vi "Manage Scan Info File.vi"(7 "CONFIGURATION CLUSTER IN":T1, 8 "SAVE MODE":enum16{"DO NOT SAVE", "SAVE .CNF FILE"}(ring), 9 "PROCESSING MODE":T3(ring), 11 "SCAN INFO CLUSTER ARRAY IN":T2(array[cluster]) {"SCAN ENABLED" items=["NO", "YES"]; "INPUT" items=["ZERO", "MEAS", "CAL"]; "RANGE" items=["NO RANGE", "2 Ohms", "20 Ohms", "200 Ohms", "2 kOhms", "20 kOhms", "200 kOhms", "2 MOhms"]; "AUTORANGE" items=["NO", "YES"]; "EXCITATION" items=["NO EXCITATION", "3 uV", "10uV", "30uV", "100uV", "300uV", "1mV", "3mV"]}) -> (1 "SCAN FILE READ INFO":string, 3 "SCAN INFO CLUSTER ARRAY OUT":T2(array[cluster])=[{"SCAN ENABLED"=0, "INPUT"=0, "RANGE"=3, "AUTORANGE"=0, "EXCITATION"=0, "STAB DELAY"=0, "AVERAGE COUNT"=1}, {"SCAN ENABLED"=0, "INPUT"=0, "RANGE"=3, "AUTORANGE"=0, "EXCITATION"=0, "STAB DELAY"=0, "AVERAGE COUNT"=1}, {"SCAN ENABLED"=0, "INPUT"=0, "RANGE"=3, "AUTORANGE"=0, "EXCITATION"=0, "STAB DELAY"=0, "AVERAGE COUNT"=1}, {"SCAN ENABLED"=0, "INPUT"=0, "RANGE"=3, "AUTORANGE"=0, "EXCITATION"=0, "STAB DELAY"=0, "AVERAGE COUNT"=1}, {"SCAN ENABLED"=0, "INPUT"=0, "RANGE"=3, "AUTORANGE"=0, "EXCITATION"=0, "STAB DELAY"=0, "AVERAGE COUNT"=1}, {"SCAN ENABLED"=0, "INPUT"=0, "RANGE"=3, "AUTORANGE"=0, "EXCITATION"=0, "STAB DELAY"=0, "AVERAGE COUNT"=1}, {"SCAN ENABLED"=0, "INPUT"=0, "RANGE"=3, "AUTORANGE"=0, "EXCITATION"=0, "STAB DELAY"=0, "AVERAGE COUNT"=1}, {"SCAN ENABLED"=0, "INPUT"=0, "RANGE"=3, "AUTORANGE"=0, "EXCITATION"=0, "STAB DELAY"=0, "AVERAGE COUNT"=1}] {"SCAN ENABLED" items=["NO", "YES"]; "INPUT" items=["ZERO", "MEAS", "CAL"]; "RANGE" items=["NO RANGE", "2 Ohms", "20 Ohms", "200 Ohms", "2 kOhms", "20 kOhms", "200 kOhms", "2 MOhms"]; "AUTORANGE" items=["NO", "YES"]; "EXCITATION" items=["NO EXCITATION", "3 uV", "10uV", "30uV", "100uV", "300uV", "1mV", "3mV"]}, 5 "CONFIGURATION CLUSTER OUT":T1)   [LabVIEW 2012]
doc: "Read, edit and save the Scan Info File.\nScan Info File specifies the settings that\nare used for each scan-enabled channel in\na scanner application."
uses:
  <vilib>/Utility/error.llb/DialogType.ctl
panel:
  in  "EDIT INFO":T2(array[cluster])=[{"SCAN ENABLED"=0, "INPUT"=0, "RANGE"=3, "AUTORANGE"=0, "EXCITATION"=0, "STAB DELAY"=0, "AVERAGE COUNT"=1}, {"SCAN ENABLED"=0, "INPUT"=0, "RANGE"=3, "AUTORANGE"=0, "EXCITATION"=0, "STAB DELAY"=0, "AVERAGE COUNT"=1}, {"SCAN ENABLED"=0, "INPUT"=0, "RANGE"=3, "AUTORANGE"=0, "EXCITATION"=0, "STAB DELAY"=0, "AVERAGE COUNT"=1}, {"SCAN ENABLED"=0, "INPUT"=0, "RANGE"=3, "AUTORANGE"=0, "EXCITATION"=0, "STAB DELAY"=0, "AVERAGE COUNT"=1}, {"SCAN ENABLED"=0, "INPUT"=0, "RANGE"=3, "AUTORANGE"=0, "EXCITATION"=0, "STAB DELAY"=0, "AVERAGE COUNT"=1}, {"SCAN ENABLED"=0, "INPUT"=0, "RANGE"=3, "AUTORANGE"=0, "EXCITATION"=0, "STAB DELAY"=0, "AVERAGE COUNT"=1}, {"SCAN ENABLED"=0, "INPUT"=0, "RANGE"=3, "AUTORANGE"=0, "EXCITATION"=0, "STAB DELAY"=0, "AVERAGE COUNT"=1}, {"SCAN ENABLED"=0, "INPUT"=0, "RANGE"=3, "AUTORANGE"=0, "EXCITATION"=0, "STAB DELAY"=0, "AVERAGE COUNT"=1}] {"SCAN ENABLED" items=["NO", "YES"]; "INPUT" items=["ZERO", "MEAS", "CAL"]; "RANGE" items=["NO RANGE", "2 Ohms", "20 Ohms", "200 Ohms", "2 kOhms", "20 kOhms", "200 kOhms", "2 MOhms"]; "AUTORANGE" items=["NO", "YES"]; "EXCITATION" items=["NO EXCITATION", "3 uV", "10uV", "30uV", "100uV", "300uV", "1mV", "3mV"]}
  in  "DISCARD":bool
  in  "ACCEPT":bool
  out "FILE READ INFO":string
  out "INFO STRING 1":string
  # "Manage Scan Info File.vi"
  # "Scan setting can be \nedited after this VI has\nbeen started  in the \n\"read and edit\" \nprocessing mode."
  # "AND PROCEED"
  # "This VI has four processing modes and two save modes:\n1. NONE:  The input Scan Info Cluster goes transparently through the VI.\n                   The cluster can be saved/not saved.\n2. READ: The  \"avs47b_scan_info.cnf\" file is read from the operating \n                   directory, and is the output of the VI.  The output cluster can\n                    be saved, but as there are no changes in this case, saving is\n                    not meaningful. If the information file is not found or is \n                    invalid, a default cluster is used instead. The default settings\n                    must be edited in order to be useful.\n3.  READ AND EDIT: The information file is read and settings for any or\n                    all of the 8 channels can be edited by selecting values in\n                    the \"SCAN INFO\" array. Once ready, choose either to accept\n                    or discard the edits and the VI proceeds to the next step,\n                    which is to save or not to save the settings, depending on\n                    the selected save mode. \n                            Because the VI stops for editing, this processing mode\n                     is not suitable for programmatic use. It can, however,  be\n                     used as such for creating an info file with useful settings.\n4. DEFAULTS:  The output is a default scan info cluster, which can be\n                      saved/not saved depending on the save settings.  The VI\n                       does not try to read the disk file."
  # "If this VI does not find the file  Avs47b_scan_info.cnf in the operating\ndirectory, it creates a default file, which you must then edit according\nto your experimental setup. Use \"Scanner with R and T displays.vi\"\nfor editing and saving the information file.\n\nThis information file specifies whether a channel is included in the\nscan cycle or not, the position of the input switch,  measuring range\n(or initial range, if autoranging is enabled),  autoranging enabled/disabled\nfor this channel, excitation, stabilisation delay and average count for\nthis channel."
  # "SCAN INFO"
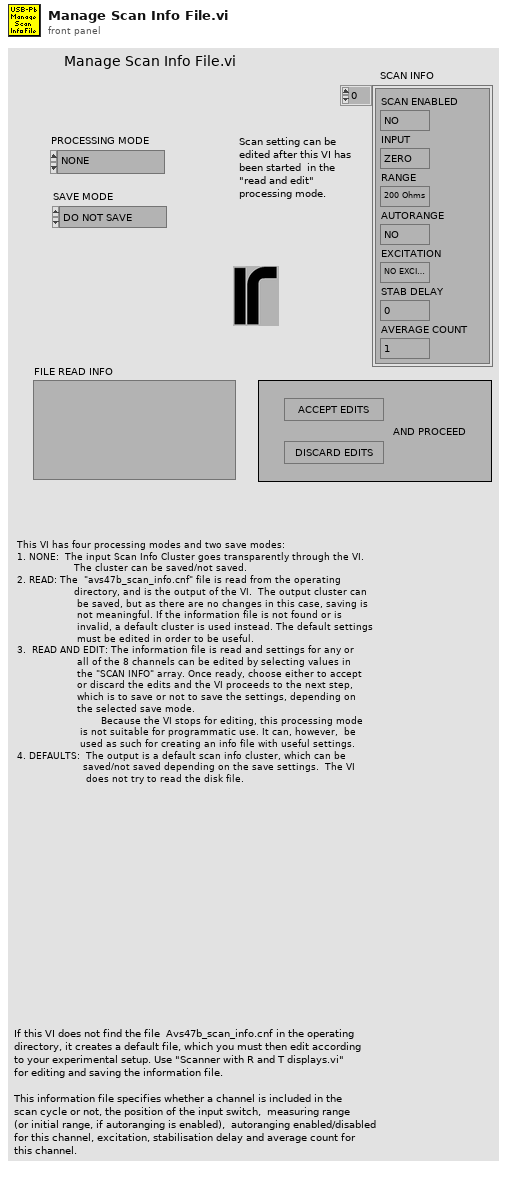
[diagram p1: front panel]
types:
  T1 = cluster{"VISA RESOURCE":refnum<visa-resource-name>, "PICOBUS ADDRESS":u8, "DISABLE AL":u8, "REMOTE":u8, "INPUT":u8, "CHANNEL":u8, "RANGE":u8, "EXCITATION":u8, "DISPLAY":u8, "DIGITAL REFERENCE":u16, "SET POINT":dbl, "PROP GAIN":u8, "INTG":u8, "DERIV":u8, "POWER BIAS":u8, "POWER RANGE":u8, "INFO STRING":string, "HEATER RESISTANCE":dbl, "INTERVAL":u8, " SENSOR dR/dT":u8}
  T2 = cluster{"SCAN ENABLED":u8, "INPUT":u8, "RANGE":u8, "AUTORANGE":u8, "EXCITATION":u8, "STAB DELAY":i32, "AVERAGE COUNT":i32}[]
  T3 = enum16{"NONE", "READ", "READ AND EDIT", "DEFAULTS"}
  T4 = cluster{"SCAN ENABLED":u8, "INPUT":u8, "RANGE":u8, "AUTORANGE":u8, "EXCITATION":u8, "STAB DELAY":i32, "AVERAGE COUNT":i32}
  T5 = enum16{"open", "replace", "create", "open or create", "replace or create", "replace or create with confirmation"}
  T6 = typedef "DialogType.ctl" = u16
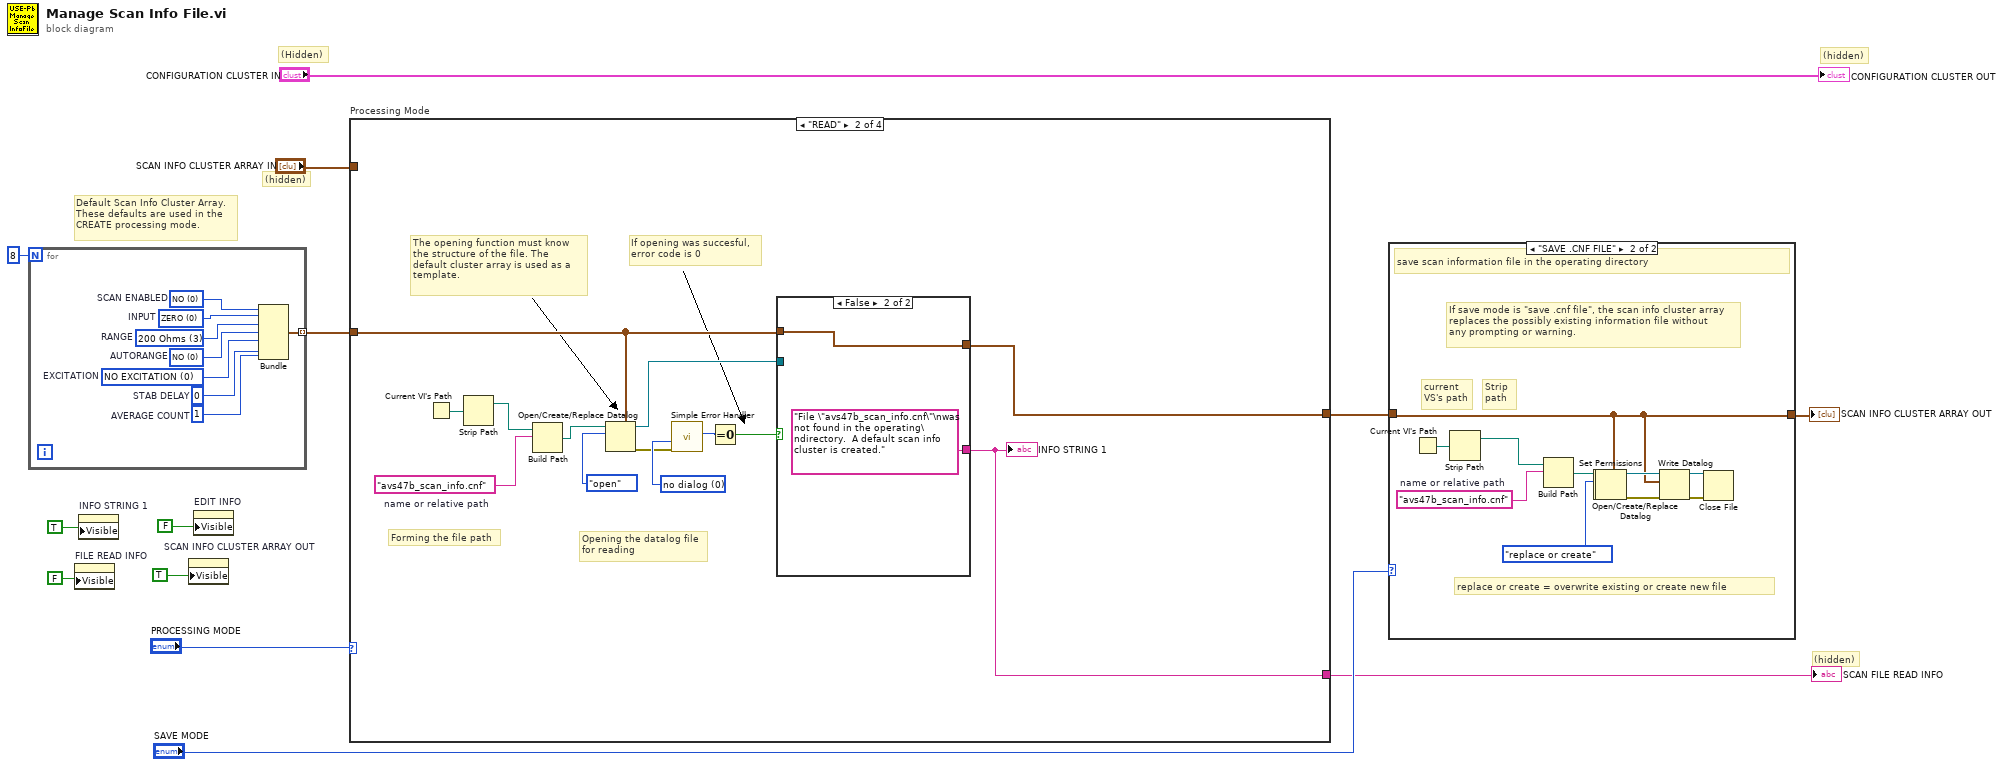
[diagram p0: block diagram]
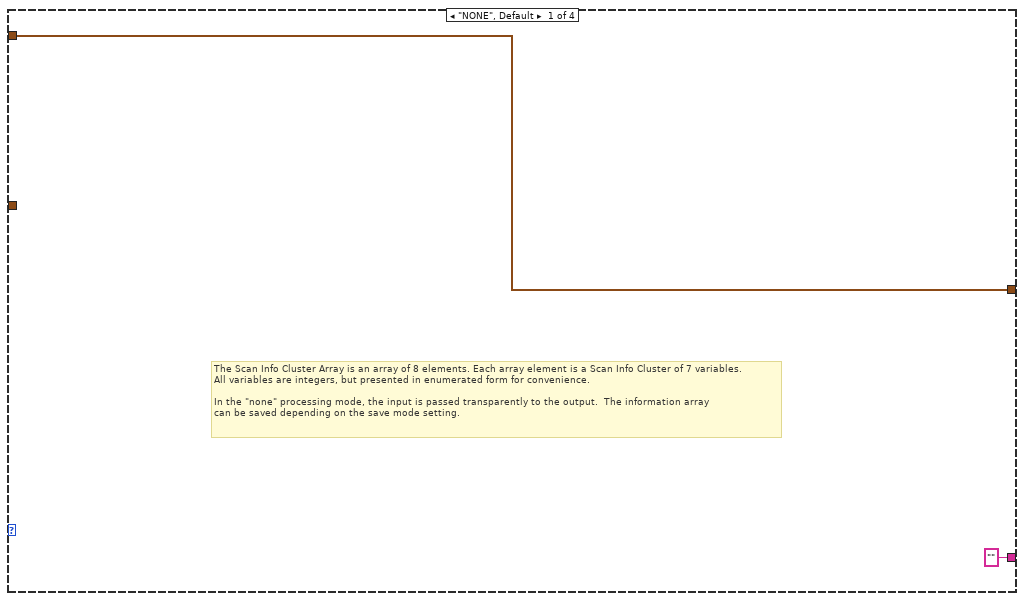
[diagram p3: hidden frame]
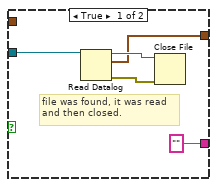
[diagram p4: hidden frame]
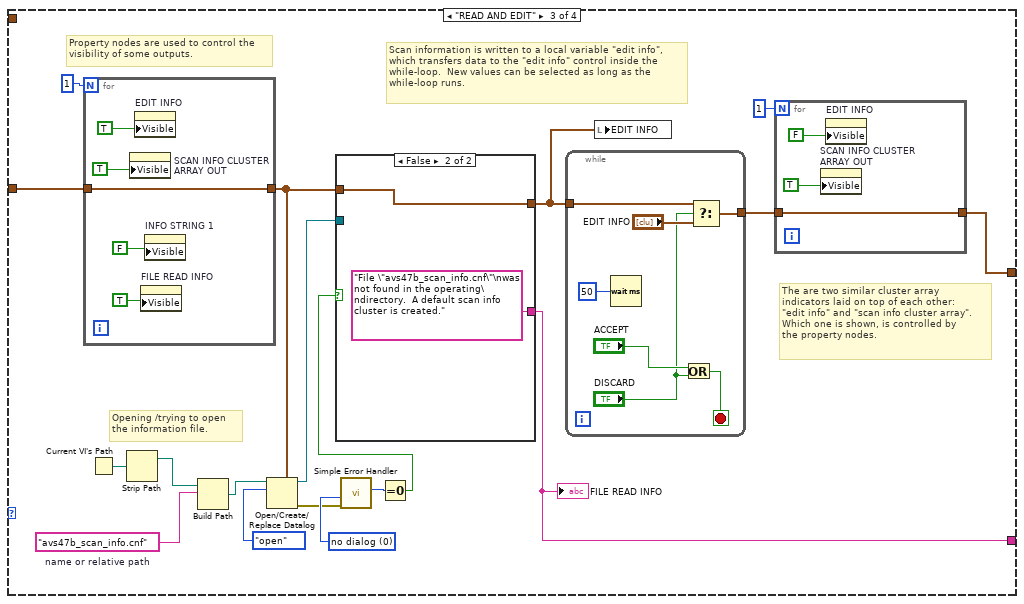
[diagram p5: hidden frame]
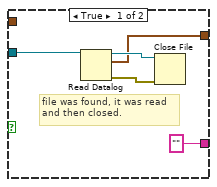
[diagram p6: hidden frame]
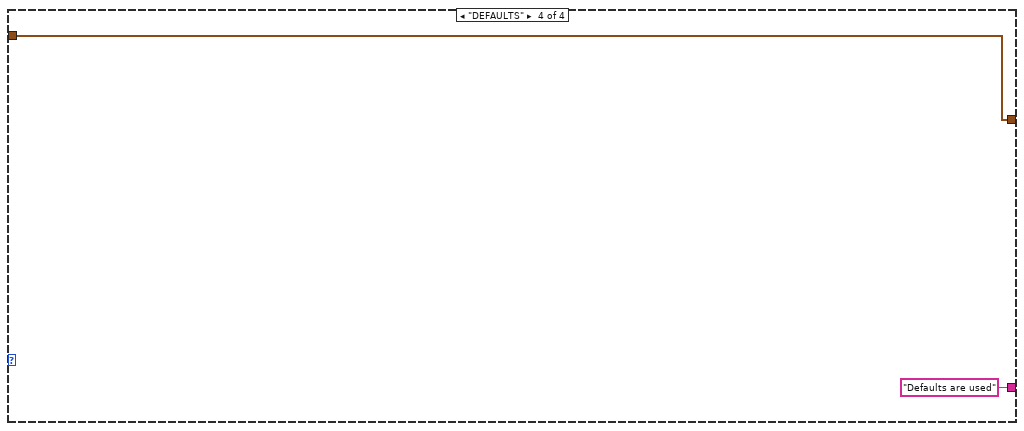
[diagram p7: hidden frame]
diagram:
  # "(Hidden)"
  # "(hidden)"
  # "(hidden)"
  # "(hidden)"
  # "Default Scan Info Cluster Array.\nThese defaults are used in the\nCREATE processing mode."
  n1 = for {
    N: 8 -> [_]
    tunnel: [w14] -> w12 mode=indexing
    w15 = 1  # AVERAGE COUNT
    w16 = 0  # STAB DELAY
    w17 = u8 0 items=["NO EXCITATION", "3 uV", "10uV", "30uV", "100uV", "300uV", "1mV", "3mV"]  # EXCITATION
    w18 = u8 0 items=["NO", "YES"]  # AUTORANGE
    w19 = u8 3 items=["NO RANGE", "2 Ohms", "20 Ohms", "200 Ohms", "2 kOhms", "20 kOhms", "200 kOhms", "2 MOhms"]  # RANGE
    w20 = u8 0 items=["ZERO", "MEAS", "CAL"]  # INPUT
    w21 = u8 0 items=["NO", "YES"]  # SCAN ENABLED
    n2 = Bundle("SCAN ENABLED"=w21, "INPUT"=w20, "RANGE"=w19, "AUTORANGE"=w18, "EXCITATION"=w17, "STAB DELAY"=w16, "AVERAGE COUNT"=w15) -> (w14:T4)  [unwired: 1 in]
  }
  n3 = property on="FILE READ INFO" class="Str"("Visible"=FALSE) -> ()  [unwired: 2 in, 2 out]
  n4 = property on="INFO STRING 1" class="Str"("Visible"=TRUE) -> ()  [unwired: 2 in, 2 out]
  n5 = property on="SCAN INFO CLUSTER ARRAY OUT" class="Arr (strict)"("Visible"=TRUE) -> ()  [unwired: 2 in, 2 out]
  n6 = property on="EDIT INFO" class="Arr (strict)"("Visible"=FALSE) -> ()  [unwired: 2 in, 2 out]
  n7 = case "Processing Mode" shown="\"READ\"" "PROCESSING MODE" {
    tunnel: w12 -> [_ w28 w50 w85]
    tunnel: "SCAN INFO CLUSTER ARRAY IN" -> [w23 _ _ _]
    tunnel: [w23 w25 w47 w85] -> w5
    tunnel: ["" w24 w44 "Defaults are used"] -> w2
    frame "NONE", Default {
      # "The Scan Info Cluster Array is an array of 8 elements. Each array element is a Scan Info Cluster of 7 variables.\nAll variables are integers, but presented in enumerated form for convenience.\n\nIn the \"none\" processing mode, the input is passed transparently to the output.  The information array\ncan be saved depending on the save mode setting."
    }
    frame "READ" {
      w34 = T6 0 items=["no dialog", "OK message", "continue or stop message", "OK message + warnings", "continue/stop + warnings"] ("type of dialog (OK msg:1)")
      w30 = "avs47b_scan_info.cnf"  # name or relative path
      # "The opening function must know\nthe structure of the file. The \ndefault cluster array is used as a \ntemplate."
      # "If opening was succesful,\nerror code is 0"
      # "Opening the datalog file\nfor reading"
      # "Forming the file path"
      n8 = Current VI's Path() -> (path=w31:path)
      n9 = Strip Path(path=w31) -> (stripped path=w32:path)  [unwired: 1 out]
      n10 = Build Path(base path=w32, name or relative path=w30) -> (appended path=w27:path)
      n11 = Open/Create/Replace Datalog(5:w28, 10:T5."open" ("operation (0:open)"), 11:w27) -> (0:w33:errorcluster, 3:w26:refnum<k1>)  [unwired: 3 in, 1 out]
      n12 = call <vilib>:"Simple Error Handler.vi"("type of dialog (OK msg:1)"=w34, "error in (no error)"=w33) -> ("code out"=w36:i32)  [unwired: 3 in, 4 out]
      n13 = Equal To 0?(x=w36) -> (x = 0?=w29:bool)
      n14 = case shown="False" w29 {
        tunnel: w28 -> [_ w43]
        tunnel: [w39 w43] -> w25
        tunnel: ["" "File \"avs47b_scan_info.cnf\"\nwas not found in the operating\ndirectory.  A default scan info cluster is created."] -> w24
        tunnel: w26 -> [w37 _]
        frame True {
          # "file was found, it was read\nand then closed."
          n15 = Read Datalog(7:w37) -> (0:w41:errorcluster, 2:w39:T2, 3:w40:refnum<k1>)  [unwired: 2 in]
          n16 = Close File(refnum=w40, error in=w41) -> ()  [unwired: 2 out]
        }
        frame False {
        }
      }
      "INFO STRING 1" <- w24
    }
    frame "READ AND EDIT" {
      w59 = T6 0 items=["no dialog", "OK message", "continue or stop message", "OK message + warnings", "continue/stop + warnings"] ("type of dialog (OK msg:1)")
      w55 = "avs47b_scan_info.cnf"  # name or relative path
      # "The are two similar cluster array\nindicators laid on top of each other:\n\"edit info\" and \"scan info cluster array\".\nWhich one is shown, is controlled by\nthe property nodes."
      # "Scan information is written to a local variable \"edit info\",\nwhich transfers data to the \"edit info\" control inside the\nwhile-loop.  New values can be selected as long as the\nwhile-loop runs."
      # "Opening /trying to open\nthe information file."
      # "Property nodes are used to control the\nvisibility of some outputs."
      n17 = for {
        N: 1 -> [_]
        tunnel: w50 -> [w67]
        tunnel: [w67] -> w49
        n18 = property on="SCAN INFO CLUSTER ARRAY OUT" class="Arr (strict)"("Visible"=TRUE) -> ()  [unwired: 2 in, 2 out]
        n19 = property on="EDIT INFO" class="Arr (strict)"("Visible"=TRUE) -> ()  [unwired: 2 in, 2 out]
        n20 = property on="FILE READ INFO" class="Str"("Visible"=TRUE) -> ()  [unwired: 2 in, 2 out]
        n21 = property on="INFO STRING 1" class="Str"("Visible"=FALSE) -> ()  [unwired: 2 in, 2 out]
      }
      n22 = Current VI's Path() -> (path=w56:path)
      n23 = Strip Path(path=w56) -> (stripped path=w57:path)  [unwired: 1 out]
      n24 = Build Path(base path=w57, name or relative path=w55) -> (appended path=w53:path)
      n25 = Open/Create/Replace Datalog(5:w49, 10:T5."open" ("operation (0:open)"), 11:w53) -> (0:w58:errorcluster, 3:w52:refnum<k1>)  [unwired: 3 in, 1 out]
      n26 = call <vilib>:"Simple Error Handler.vi"("type of dialog (OK msg:1)"=w59, "error in (no error)"=w58) -> ("code out"=w61:i32)  [unwired: 3 in, 4 out]
      n27 = Equal To 0?(x=w61) -> (x = 0?=w54:bool)
      n28 = case shown="False" w54 {
        tunnel: w49 -> [_ w83]
        tunnel: [w79 w83] -> w51
        tunnel: ["" "File \"avs47b_scan_info.cnf\"\nwas not found in the operating\ndirectory.  A default scan info cluster is created."] -> w44
        tunnel: w52 -> [w77 _]
        frame True {
          # "file was found, it was read\nand then closed."
          n29 = Read Datalog(7:w77) -> (0:w81:errorcluster, 2:w79:T2, 3:w80:refnum<k1>)  [unwired: 2 in]
          n30 = Close File(refnum=w80, error in=w81) -> ()  [unwired: 2 out]
        }
        frame False {
        }
      }
      "FILE READ INFO" <- w44
      n31 = while {
        tunnel: w51 -> [w73]
        tunnel: [w70] -> w48
        stop <- w74 stop-if-true
        n32 = Wait (ms)(milliseconds to wait=u32 50) -> ()  [unwired: 1 out]
        n33 = Or(x="ACCEPT", y="DISCARD") -> (x .or. y?=w74:bool)
        n34 = Select(t=w73, s="DISCARD", f="EDIT INFO") -> (s? t:f=w70:T2)
      }
      n35 = local write "EDIT INFO"(w51) -> ()
      n36 = for {
        N: 1 -> [_]
        tunnel: w48 -> [w62]
        tunnel: [w62] -> w47
        n37 = property on="SCAN INFO CLUSTER ARRAY OUT" class="Arr (strict)"("Visible"=TRUE) -> ()  [unwired: 2 in, 2 out]
        n38 = property on="EDIT INFO" class="Arr (strict)"("Visible"=FALSE) -> ()  [unwired: 2 in, 2 out]
      }
    }
    frame "DEFAULTS" {
    }
  }
  "SCAN FILE READ INFO" <- w2
  n39 = case shown="\"SAVE .CNF FILE\"" "SAVE MODE" {
    tunnel: [w86 w87] -> w4
    tunnel: w5 -> [w86 w87]
    frame "DO NOT SAVE", Default {
      # "do not save nor create configuration file"
    }
    frame "SAVE .CNF FILE" {
      w92 = "avs47b_scan_info.cnf"  # name or relative path
      # "If save mode is \"save .cnf file\", the scan info cluster array\nreplaces the possibly existing information file without \nany prompting or warning."
      # "Strip\npath"
      # "current\nVS's path"
      # "replace or create = overwrite existing or create new file"
      # "save scan information file in the operating directory"
      n40 = Current VI's Path() -> (path=w94:path)
      n41 = Strip Path(path=w94) -> (stripped path=w95:path)  [unwired: 1 out]
      n42 = Build Path(base path=w95, name or relative path=w92) -> (appended path=w93:path)
      n43 = Open/Create/Replace Datalog(5:w87, 10:T5."replace or create" ("operation (0:open)"), 11:w93) -> (0:w96:errorcluster, 3:w88:refnum<k1>)  [unwired: 3 in, 1 out]
      n44 = Set Permissions(8:w96, 11:w93) -> (0:w89:errorcluster)  [unwired: 3 in, 1 out]
      n45 = Write Datalog(4:w89, 6:w87, 7:w88) -> (0:w91:errorcluster, 3:w90:refnum<k1>)
      n46 = Close File(refnum=w90, error in=w91) -> ()  [unwired: 2 out]
    }
  }
  "SCAN INFO CLUSTER ARRAY OUT" <- w4
  "CONFIGURATION CLUSTER OUT" <- "CONFIGURATION CLUSTER IN"
